vi "SCP_Message_Selection.vi"(11 "SCP_Cluster_In":T1) -> (2 "SCP_Command_String_Out":string, 3 "SCP_Cluster_Out":T1)   [LabVIEW 2018, in "SCP.lvlib"]
uses:
  SCP.lvlib
  Engine/Type/SCP_Cluster.ctl
  SCP_Command_Strings.ctl
  Selection.ctl
panel:
  in  "search string":string="/home/philip/Vires21/VTD.2.1/Data/Projects/SampleProject/Scenarios/traffic_demo.xml"
  in  "SCP Commands":T2=["<SimCtrl><Start tMax=\"0\" mode=\"operation\" /></SimCtrl>", "<SimCtrl><Stop /></SimCtrl>", "<SimCtrl><Pause /></SimCtrl>", "<SimCtrl><Restart /></SimCtrl>", "<SimCtrl><Step size=\"1\" /></SimCtrl>", "<SimCtrl><Stop /></SimCtrl>\n<SimCtrl><LoadScenario filename=\"/home/philip/Vires21/VTD.2.1/Data/Projects/SampleProject/Scenarios/traffic_demo.xml\" /><Start mode=\"operation\" /></SimCtrl>"]
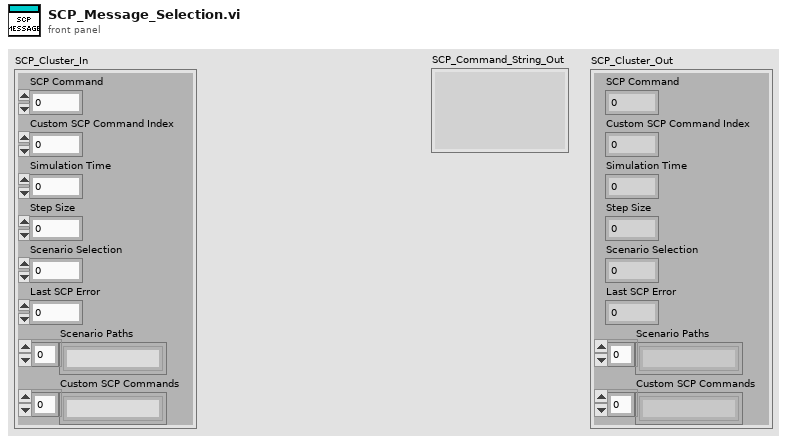
[diagram p1: front panel]
types:
  T1 = typedef "SCP.lvlib/SCP_Cluster.ctl" = cluster{"SCP Command ":i32, "Custom SCP Command Index":i32, "Simulation Time":i32, "Step Size":i32, "Scenario Selection":i32, "Last SCP Error":i32, "Scenario Paths":string[], "Custom SCP Commands":string[]}
  T2 = typedef "SCP.lvlib/SCP_Command_Strings.ctl" = string[]
  T3 = typedef "SCP.lvlib/Selection.ctl" = enum16{"Idle", "Start", "Stop", "Pause", "Restart", "Step", "Change Scenario", "Custom SCP command"}
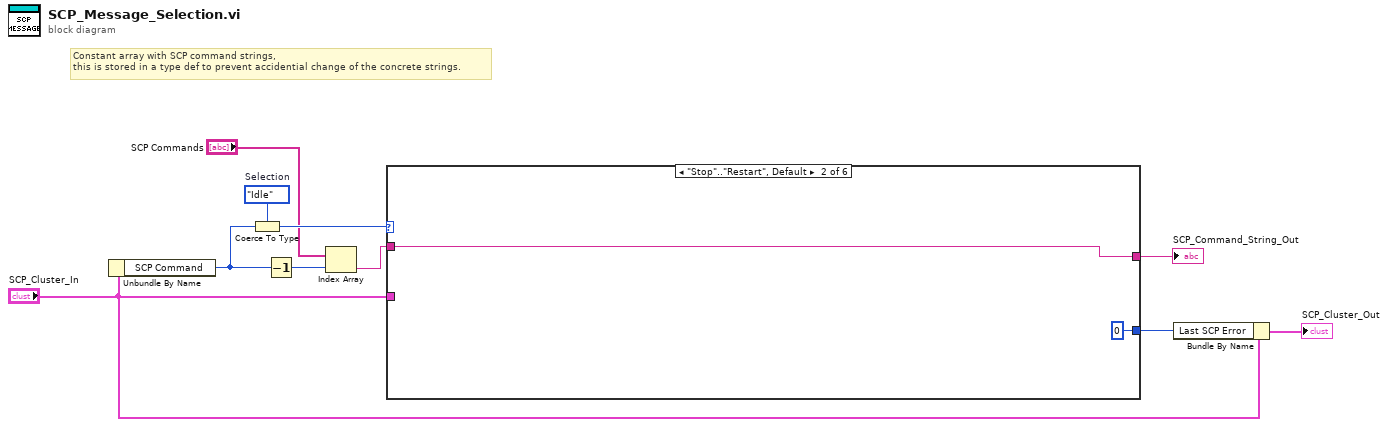
[diagram p0: block diagram]
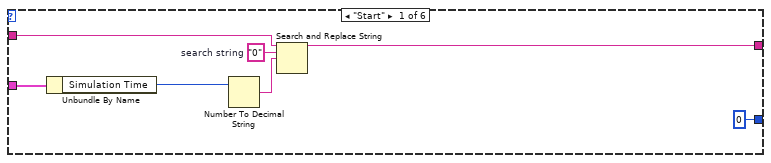
[diagram p2: hidden frame]
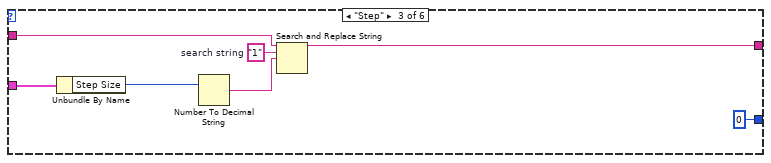
[diagram p3: hidden frame]
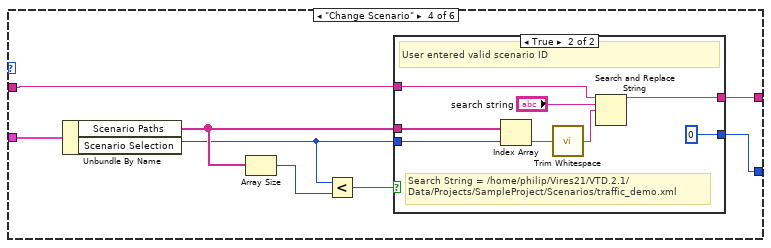
[diagram p4: hidden frame]
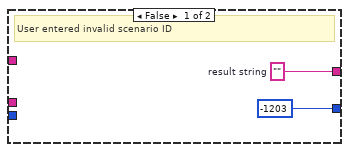
[diagram p5: hidden frame]
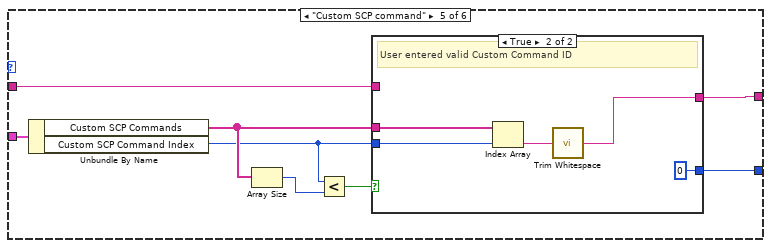
[diagram p6: hidden frame]
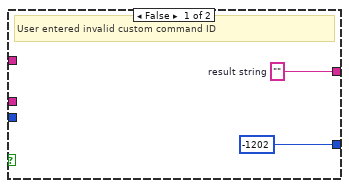
[diagram p7: hidden frame]
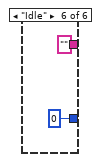
[diagram p8: hidden frame]
diagram:
  w8 = Selection."Idle"  # Selection
  # "Constant array with SCP command strings,\nthis is stored in a type def to prevent accidential change of the concrete strings."
  n1 = Unbundle By Name("SCP_Cluster_In") -> ("SCP Command"=w7:i32)
  n2 = Coerce To Type(0:w7, 1:w8) -> (2:w6:T3)
  n3 = Decrement(x=w7) -> (x-1=w4:i32)
  n4 = Index Array(array="SCP Commands", index=w4) -> (element=w9:string)
  n5 = case shown="\"Stop\"..\"Restart\", Default" w6 {
    tunnel: [w16 w19 w24 w33 w51 ""] -> w10
    tunnel: w9 -> [w17 w19 w23 w34 w50 _]
    tunnel: "SCP_Cluster_In" -> [w12 _ w21 w30 w46 _]
    tunnel: [0 0 0 w27 w45 0] -> w1
    frame "Start" {
      w15 = "0"  # search string
      n6 = Unbundle By Name(w12) -> ("Simulation Time"=w13:i32)
      n7 = Number To Decimal String(number=w13) -> (decimal integer string=w14:string)  [unwired: 1 in]
      n8 = Search and Replace String(input string=w17, search string=w15, replace string=w14) -> (result string=w16:string)  [unwired: 5 in, 3 out]
    }
    frame "Stop".."Restart", Default {
    }
    frame "Step" {
      w26 = "1"  # search string
      n9 = Unbundle By Name(w21) -> ("Step Size"=w22:i32)
      n10 = Number To Decimal String(number=w22) -> (decimal integer string=w25:string)  [unwired: 1 in]
      n11 = Search and Replace String(input string=w23, search string=w26, replace string=w25) -> (result string=w24:string)  [unwired: 5 in, 3 out]
    }
    frame "Change Scenario" {
      n12 = Unbundle By Name(w30) -> ("Scenario Paths"=w32:string[], "Scenario Selection"=w28:i32)
      n13 = Array Size(array=w32) -> (size(s)=w29:i32)
      n14 = Less?(x=w28, y=w29) -> (x < y?=w31:bool)
      n15 = case shown="True" w31 {
        tunnel: w34 -> [_ w43]
        tunnel: [w36 w42] -> w33
        tunnel: w32 -> [_ w39]
        tunnel: w28 -> [_ w38]
        tunnel: [-1203 0] -> w27
        frame False {
          w36 = ""  # result string
          # "User entered invalid scenario ID"
        }
        frame True {
          # "Search String = /home/philip/Vires21/VTD.2.1/\nData/Projects/SampleProject/Scenarios/traffic_demo.xml"
          # "User entered valid scenario ID"
          n16 = Index Array(array=w39, index=w38) -> (element=w40:string)
          n17 = call <vilib>:"Trim Whitespace.vi"("string"=w40) -> ("trimmed string"=w41:string)  [unwired: 1 in]
          n18 = Search and Replace String(input string=w43, search string="search string", replace string=w41) -> (result string=w42:string)  [unwired: 5 in, 3 out]
        }
      }
    }
    frame "Custom SCP command" {
      n19 = Unbundle By Name(w46) -> ("Custom SCP Commands"=w49:string[], "Custom SCP Command Index"=w47:i32)
      n20 = Array Size(array=w49) -> (size(s)=w48:i32)
      n21 = Less?(x=w47, y=w48) -> (x < y?=w52:bool)
      n22 = case shown="True" w52 {
        tunnel: w50 -> [_ _]
        tunnel: [w54 w56] -> w51
        tunnel: w49 -> [_ w58]
        tunnel: w47 -> [_ w57]
        tunnel: [-1202 0] -> w45
        frame False {
          w54 = ""  # result string
          # "User entered invalid custom command ID"
        }
        frame True {
          # "User entered valid Custom Command ID"
          n23 = Index Array(array=w58, index=w57) -> (element=w59:string)
          n24 = call <vilib>:"Trim Whitespace.vi"("string"=w59) -> ("trimmed string"=w56:string)  [unwired: 1 in]
        }
      }
    }
    frame "Idle" {
    }
  }
  "SCP_Command_String_Out" <- w10
  n25 = Bundle By Name(cluster="SCP_Cluster_In", "Last SCP Error"=w1) -> (→"SCP_Cluster_Out":T1)
